vi "Write Weather Forecast Data.vi"(8 "error in (no error)":errorcluster, 10 "Weather Forecast Data":refnum<vi>, 11 "Weather in":refnum<class "Weather.lvclass">) -> (0 "error out":errorcluster, 3 "Weather out":refnum<class "Weather.lvclass">)   [LabVIEW 2025, in "Weather Actor.lvlib" / "Weather.lvclass"]
uses:
  Weather.lvclass
  Weather.lvclass/Weather.ctl
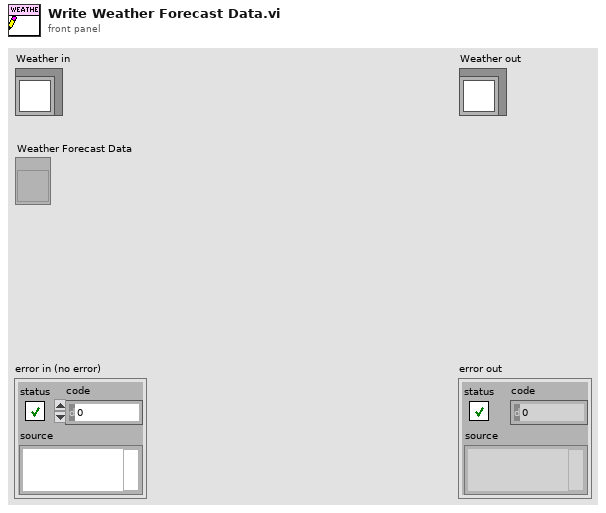
[diagram p1: front panel]
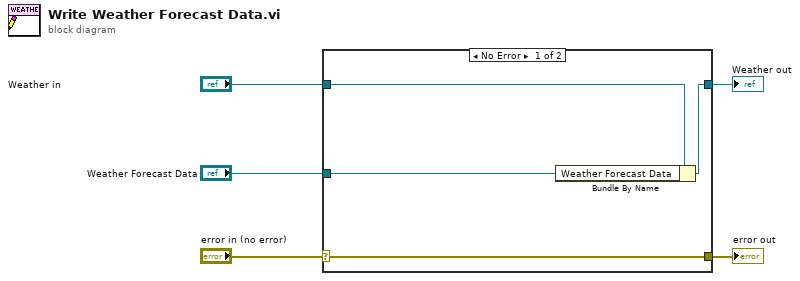
[diagram p0: block diagram]
diagram:
  n1 = case shown="No Error" "error in (no error)" {
    selector: "error in (no error)" -> [w9 w10]
    tunnel: [w9 w10] -> w4
    tunnel: [w7 w11] -> w2
    tunnel: "Weather in" -> [w8 w11]
    tunnel: "Weather Forecast Data" -> [w6 _]
    frame No Error {
      n2 = Bundle By Name(cluster=w8, "Weather Forecast Data"=w6) -> (w7:refnum<class "Weather.lvclass">)
    }
    frame Error {
    }
  }
  "error out" <- w4
  "Weather out" <- w2
